vi "Teleop.vi"(10 "Match Info":T1={"Autonomous Elapsed Seconds"=0.0, "TeleOp Elapsed Seconds"=0.0, "Disabled Elapsed Seconds"=0.0, "Visited Autonomous"=FALSE, "Visited TeleOp"=FALSE, "Visited Disabled"=FALSE, "Autonomous Settings"={"Autonomous Style"=enum."Independent", "VI Refnum"=refnum}}, 11 "Call Context":T2) -> ()   [LabVIEW 2019]
doc: "This VI is called for each TeleOp packet received from the DS where the robot is not disabled. It is often used to read from the joysticks and update I/O or to update setpoints for timed control loops. It should complete and return within 20 milliseconds or it may miss DS packets."
uses:
  <vilib>/Rock Robotics/WPI/DriverStation/WPI_DriverStationDerivedRobotMode.ctl
  <vilib>/Rock Robotics/WPI/DriverStation/WPI_DriverStationMatch Info.ctl
  <vilib>/Rock Robotics/WPI/Utilities/WPI_GetSetVariantRefNum.vi
  Robot Global Data.vi
  <vilib>/Rock Robotics/Network Tables/NT Write Number.vi
  <vilib>/Rock Robotics/WPI/DriverStation/WPI_DriverStationRobotMode2.ctl
  <vilib>/Rock Robotics/Network Tables/NT Write Numeric Array.vi
  <vilib>/Rock Robotics/WPI/RobotDrive/WPI_RobotDriveArcadeDrive_Standard(NoSaturation).vi
  <vilib>/Rock Robotics/Network Tables/NT Write Boolean.vi
panel:
  in  "error in":errorcluster
  out "interpolation value":dbl format="%0.2f"
  # "Click here to set min"
  # "Click here to set max"
  # "Click here to set min"
  # "Click here to set max"
  # "Click here to set min"
  # "Click here to set max"
  # "Click here to set min"
  # "Click here to set max"
  # "Click here to set min"
  # "Click here to set max"
  # "Click here to set min"
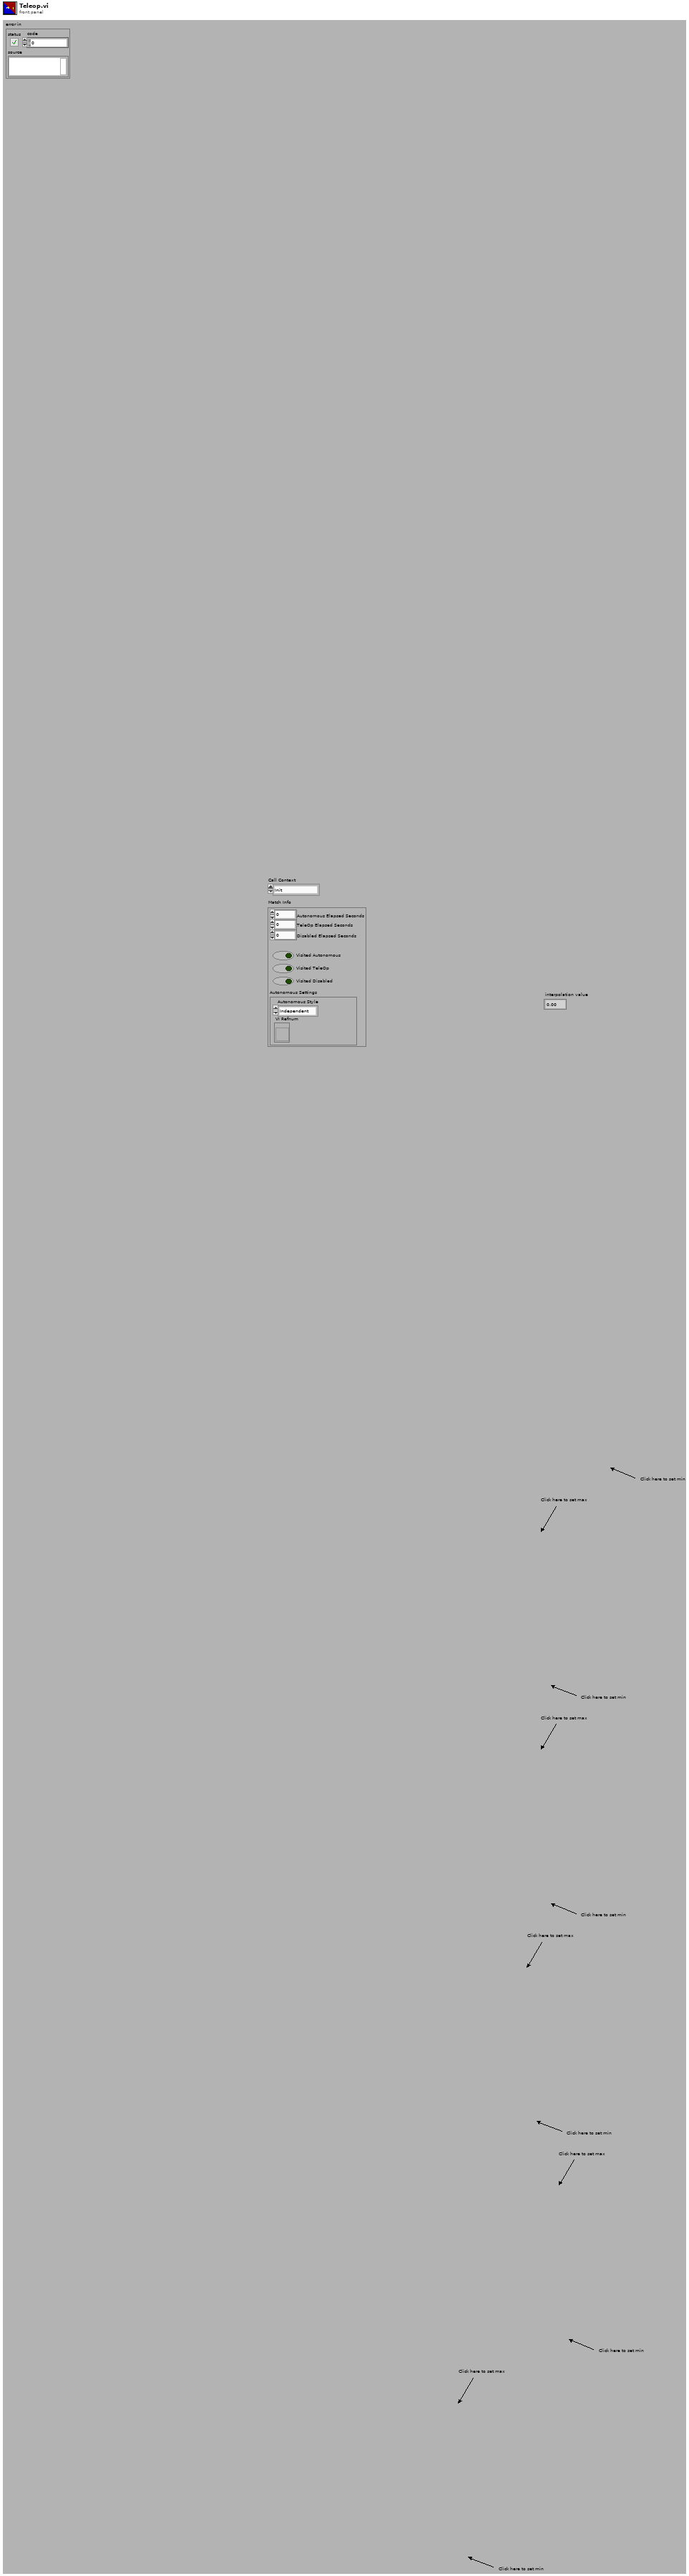
[diagram p1: front panel]
types:
  T1 = typedef "WPI_DriverStationMatch Info.ctl" = cluster{"Autonomous Elapsed Seconds":dbl, "TeleOp Elapsed Seconds":dbl, "Disabled Elapsed Seconds":dbl, "Visited Autonomous":bool, "Visited TeleOp":bool, "Visited Disabled":bool, "Autonomous Settings":cluster{"Autonomous Style":enum16{"Iterative", "Independent"}, "VI Refnum":refnum<vi>}}
  T2 = typedef "WPI_DriverStationDerivedRobotMode.ctl" = enum16{"Init", "Execute", "Stop"}
  T3 = typedef "WPI_JoystickDevRef.ctl" = cluster{"Device":T4}
  T4 = typedef "WPI_JoystickDeviceEnum.ctl" = enum16{"USB 0", "USB 1", "USB 2", "USB 3", "USB 4", "USB 5"}
  T5 = typedef "WPI_RobotDriveDevRef.ctl" = cluster{"DevStatus":errorcluster, "Motors[]":T6[], "Square Inputs":bool, "Max Output":dbl}
  T6 = typedef "WPI_MotorControlDeviceRef.ctl" = cluster{"DeviceStatus":errorcluster, "Type":T7, "PWM":cluster{"PWM Channel":T8, "DeadBand":T9}, "CAN":cluster{"Device Number":u8, "SetOutput VI Ref":variant, "GetOutput VI Ref":variant, "Enable VI Ref":variant, "Disable VI Ref":variant, "Data":variant}, "Invert":bool, "DIO PWM":cluster{"PWM \"Enable\" Channel":T8, "DIOChannel":T10, "PWM Rate":dbl}}
  T7 = typedef "WPI_MotorControlType.ctl" = enum16{"PWM", "CAN", "DIO PWM"}
  T8 = typedef "FPGA_DIOPWMChannel.ctl" = enum8{"PWM 0", "PWM 1", "PWM 2", "PWM 3", "PWM 4", "PWM 5", "PWM 6", "PWM 7", "PWM 8", "PWM 9", "PWM MXP 0", "PWM MXP 1", "PWM MXP 2", "PWM MXP 3", "PWM MXP 4", "PWM MXP 5", "PWM MXP 6", "PWM MXP 7", "PWM MXP 8", "PWM MXP 9", "Invalid"}
  T9 = typedef "WPI_PWMDeadband.ctl" = cluster{"Name":string, "maxPositivePwm":i32, "minPositivePwm":i32, "centerPwm":i32, "maxNegativePwm":i32, "minNegativePwm":i32, "angularRange":u16}
  T10 = typedef "FPGA_DIOChannel.ctl" = enum8{"DIO 0", "DIO 1", "DIO 2", "DIO 3", "DIO 4", "DIO 5", "DIO 6", "DIO 7", "DIO 8", "DIO 9", "DIO MXP 0", "DIO MXP 1", "DIO MXP 2", "DIO MXP 3", "DIO MXP 4", "DIO MXP 5", "DIO MXP 6", "DIO MXP 7", "DIO MXP 8", "DIO MXP 9", "DIO MXP 10", "DIO MXP 11", "DIO MXP 12", "DIO MXP 13", "DIO MXP 14", "DIO MXP 15", "SPI Port CS1", "SPI Port CS2", "SPI Port CS3", "SPI Port MISO", "SPI Port MOSI", "Invalid"}
  T11 = cluster{"JoystickDevRef":T3, "RobotDriveDevRef":T5}
  T12 = typedef "WPI_ServoDeviceRef.ctl" = cluster{"DeviceStatus":errorcluster, "PWM Channel":T8, "DeadBand":T9}
  T13 = typedef "WPI_DriverStationRobotMode2.ctl" = enum16{"Autonomous Disabled", "Autonomous Enabled", "Teleop Disabled", "Teleop Enabled", "Disconnected", "Finish", "Test Disabled", "Test Enabled", "Emergency Stopped"}
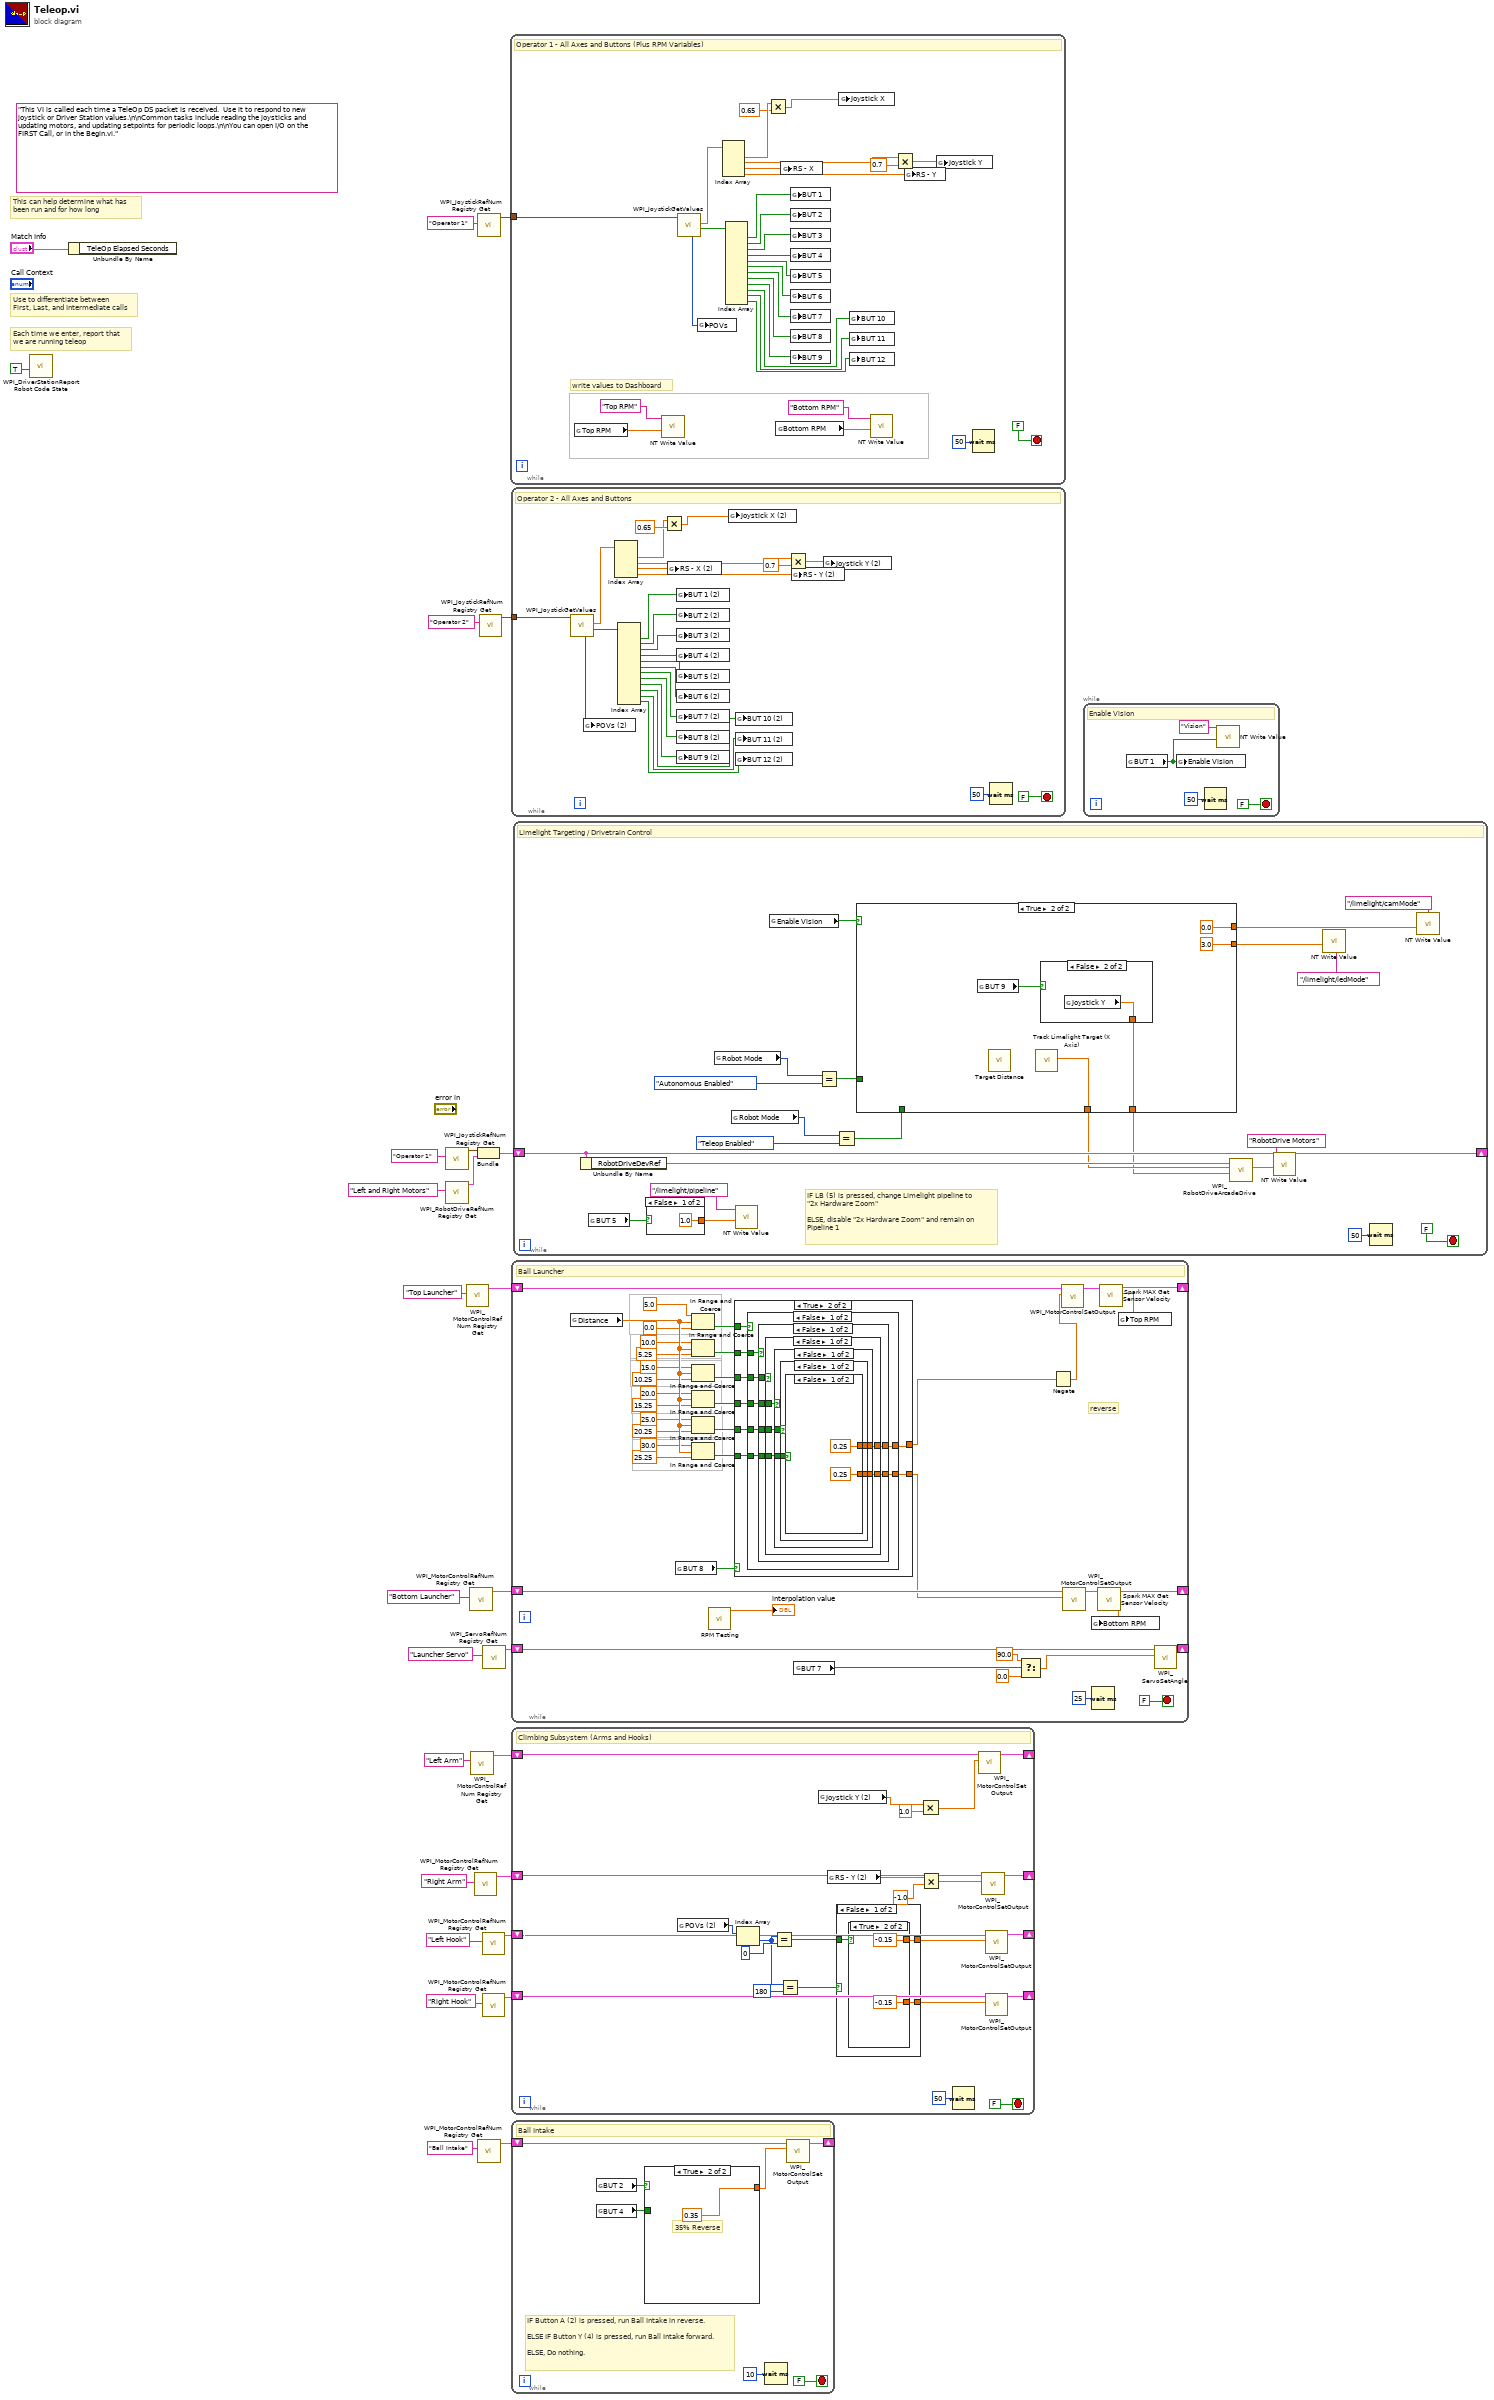
[diagram p0: block diagram]
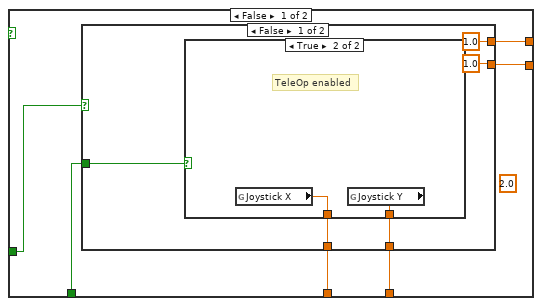
[diagram p2: hidden frame]
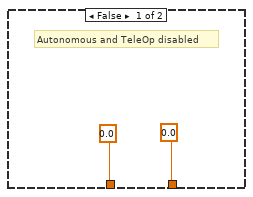
[diagram p3: hidden frame]
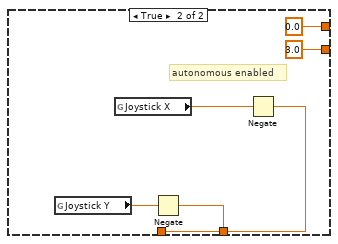
[diagram p4: hidden frame]
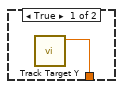
[diagram p5: hidden frame]
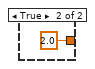
[diagram p6: hidden frame]
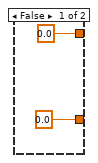
[diagram p7: hidden frame]
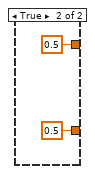
[diagram p8: hidden frame]
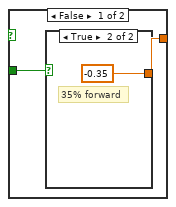
[diagram p9: hidden frame]
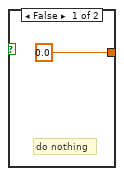
[diagram p10: hidden frame]
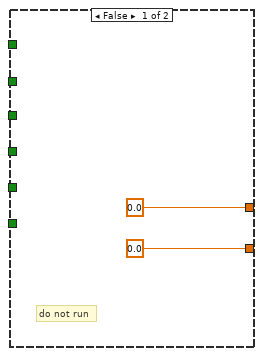
[diagram p11: hidden frame]
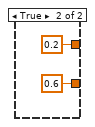
[diagram p12: hidden frame]
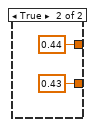
[diagram p13: hidden frame]
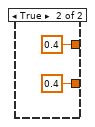
[diagram p14: hidden frame]
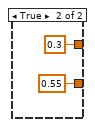
[diagram p15: hidden frame]
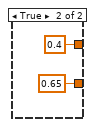
[diagram p16: hidden frame]
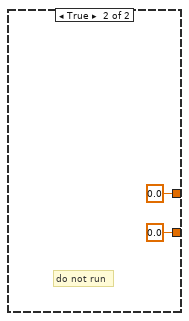
[diagram p17: hidden frame]
diagram:
  (unwired) "This VI is called each time a TeleOp DS packet is received.  Use it to respond to new joystick or Driver Station values.\n\nCommon tasks include reading the joysticks and updating motors, and updating setpoints for periodic loops.\n\nYou can open I/O on the FIRST Call, or in the Begin.vi."
  # "Each time we enter, report that\nwe are running teleop"
  # "Use to differentiate between\nFirst, Last, and Intermediate calls"
  # "This can help determine what has\nbeen run and for how long"
  n1 = call <vilib>:"WPI_DriverStationReport Robot Code State.vi"("TeleOp"=TRUE ("Autonomous")) -> ()  [unwired: 10 in, 1 out]
  n2 = Unbundle By Name("Match Info") -> ()  [unwired: 1 out]
  n3 = call <vilib>:"WPI_JoystickRefNum Registry Get.vi"("refnum name"="Operator 1") -> ("JoystickDevRef"=w3:T3)  [unwired: 1 in, 9 out]
  n4 = call <vilib>:"WPI_RobotDriveRefNum Registry Get.vi"("refnum name"="Left and Right Motors") -> ("RobotDriveDevRef"=w2:T5)  [unwired: 1 in, 9 out]
  n5 = call <vilib>:"WPI_MotorControlRefNum Registry Get.vi"("refnum name"="Top Launcher") -> ("MotorControlDevRef"=w21:T6)  [unwired: 9 in, 1 out]
  n6 = call <vilib>:"WPI_MotorControlRefNum Registry Get.vi"("refnum name"="Bottom Launcher") -> ("MotorControlDevRef"=w23:T6)  [unwired: 9 in, 1 out]
  n7 = call <vilib>:"WPI_MotorControlRefNum Registry Get.vi"("refnum name"="Left Arm") -> ("MotorControlDevRef"=w15:T6)  [unwired: 9 in, 1 out]
  n8 = call <vilib>:"WPI_MotorControlRefNum Registry Get.vi"("refnum name"="Right Arm") -> ("MotorControlDevRef"=w14:T6)  [unwired: 9 in, 1 out]
  n9 = Bundle("JoystickDevRef"=w3, "RobotDriveDevRef"=w2) -> (w1:T11)  [unwired: 1 out]
  n10 = call <vilib>:"WPI_JoystickRefNum Registry Get.vi"("refnum name"="Operator 1") -> ("JoystickDevRef"=w6:T3)  [unwired: 1 in, 9 out]
  n11 = call <vilib>:"WPI_MotorControlRefNum Registry Get.vi"("refnum name"="Ball Intake") -> ("MotorControlDevRef"=w17:T6)  [unwired: 9 in, 1 out]
  n12 = call <vilib>:"WPI_JoystickRefNum Registry Get.vi"("refnum name"="Operator 2") -> ("JoystickDevRef"=w7:T3)  [unwired: 1 in, 9 out]
  n13 = call <vilib>:"WPI_MotorControlRefNum Registry Get.vi"("refnum name"="Left Hook") -> ("MotorControlDevRef"=w12:T6)  [unwired: 9 in, 1 out]
  n14 = call <vilib>:"WPI_MotorControlRefNum Registry Get.vi"("refnum name"="Right Hook") -> ("MotorControlDevRef"=w11:T6)  [unwired: 9 in, 1 out]
  n15 = call <vilib>:"WPI_ServoRefNum Registry Get.vi"("refnum name"="Launcher Servo") -> ("ServoDeviceRef"=w19:T12)  [unwired: 9 in, 1 out]
  n16 = while {
    tunnel: w6 -> [w28]
    stop <- FALSE stop-if-true
    # "write values to Dashboard"
    # "Operator 1 - All Axes and Buttons (Plus RPM Variables)"
    n17 = global read "Robot Global Data.vi" "Top RPM"() -> (w39:dbl)
    n18 = call-poly <vilib>:"NT Write Value.vi"("Numeric"=w39, "Name"="Top RPM") -> ()  [unwired: 9 in, 1 out]
    n19 = call <vilib>:"WPI_JoystickGetValues.vi"("JoystickDevRef"=w28) -> ("Buttons"=w56:bool[], "Axes"=w43:dbl[], "POVs"=w35:i16[])  [unwired: 6 in, 2 out]
    n20 = global write "Robot Global Data.vi" "POVs"(w35) -> ()
    n21 = Index Array(array=w43) -> (element #1=w32:dbl, element #2=w34:dbl, element #3=w36:dbl, element #4=w42:dbl)  [unwired: 4 in]
    n22 = Index Array(array=w56) -> (element #1=w55:bool, element #2=w54:bool, element #3=w53:bool, element #4=w52:bool, element #5=w51:bool, element #6=w50:bool, element #7=w49:bool, element #8=w48:bool, element #9=w47:bool, element #10=w46:bool, element #11=w45:bool, element #12=w44:bool)  [unwired: 12 in]
    n23 = Multiply(x=w32, y=0.65) -> (x*y=w33:dbl)
    n24 = global read "Robot Global Data.vi" "Bottom RPM"() -> (w37:dbl)
    n25 = global write "Robot Global Data.vi" "RS - X"(w36) -> ()
    n26 = global write "Robot Global Data.vi" "BUT 1"(w55) -> ()
    n27 = global write "Robot Global Data.vi" "BUT 2"(w54) -> ()
    n28 = global write "Robot Global Data.vi" "BUT 3"(w53) -> ()
    n29 = global write "Robot Global Data.vi" "BUT 4"(w52) -> ()
    n30 = global write "Robot Global Data.vi" "BUT 5"(w51) -> ()
    n31 = global write "Robot Global Data.vi" "BUT 6"(w50) -> ()
    n32 = global write "Robot Global Data.vi" "BUT 7"(w49) -> ()
    n33 = global write "Robot Global Data.vi" "BUT 8"(w48) -> ()
    n34 = global write "Robot Global Data.vi" "BUT 9"(w47) -> ()
    n35 = global write "Robot Global Data.vi" "Joystick X"(w33) -> ()
    n36 = global write "Robot Global Data.vi" "BUT 10"(w46) -> ()
    n37 = global write "Robot Global Data.vi" "BUT 11"(w45) -> ()
    n38 = global write "Robot Global Data.vi" "BUT 12"(w44) -> ()
    n39 = call-poly <vilib>:"NT Write Value.vi"("Numeric"=w37, "Name"="Bottom RPM") -> ()  [unwired: 9 in, 1 out]
    n40 = Multiply(x=w34, y=0.7) -> (x*y=w30:dbl)
    n41 = global write "Robot Global Data.vi" "RS - Y"(w42) -> ()
    n42 = global write "Robot Global Data.vi" "Joystick Y"(w30) -> ()
    n43 = Wait (ms)(milliseconds to wait=u32 50) -> ()  [unwired: 1 out]
  }
  n44 = while {
    tunnel: w7 -> [w58]
    stop <- FALSE stop-if-true
    # "Operator 2 - All Axes and Buttons"
    n45 = call <vilib>:"WPI_JoystickGetValues.vi"("JoystickDevRef"=w58) -> ("Buttons"=w60:bool[], "Axes"=w73:dbl[], "POVs"=w59:i16[])  [unwired: 6 in, 2 out]
    n46 = global write "Robot Global Data.vi" "POVs (2)"(w59) -> ()
    n47 = Index Array(array=w73) -> (element #1=w78:dbl, element #2=w76:dbl, element #3=w75:dbl, element #4=w74:dbl)  [unwired: 4 in]
    n48 = Index Array(array=w60) -> (element #1=w61:bool, element #2=w62:bool, element #3=w63:bool, element #4=w64:bool, element #5=w65:bool, element #6=w66:bool, element #7=w67:bool, element #8=w68:bool, element #9=w69:bool, element #10=w70:bool, element #11=w71:bool, element #12=w72:bool)  [unwired: 12 in]
    n49 = Multiply(x=w78, y=0.65) -> (x*y=w77:dbl)
    n50 = global write "Robot Global Data.vi" "RS - X (2)"(w75) -> ()
    n51 = global write "Robot Global Data.vi" "BUT 1 (2)"(w61) -> ()
    n52 = global write "Robot Global Data.vi" "BUT 2 (2)"(w62) -> ()
    n53 = global write "Robot Global Data.vi" "BUT 3 (2)"(w63) -> ()
    n54 = global write "Robot Global Data.vi" "BUT 4 (2)"(w64) -> ()
    n55 = global write "Robot Global Data.vi" "BUT 5 (2)"(w65) -> ()
    n56 = global write "Robot Global Data.vi" "BUT 6 (2)"(w66) -> ()
    n57 = global write "Robot Global Data.vi" "BUT 7 (2)"(w67) -> ()
    n58 = global write "Robot Global Data.vi" "BUT 8 (2)"(w68) -> ()
    n59 = global write "Robot Global Data.vi" "BUT 9 (2)"(w69) -> ()
    n60 = global write "Robot Global Data.vi" "Joystick X (2)"(w77) -> ()
    n61 = global write "Robot Global Data.vi" "BUT 10 (2)"(w70) -> ()
    n62 = global write "Robot Global Data.vi" "BUT 11 (2)"(w71) -> ()
    n63 = global write "Robot Global Data.vi" "BUT 12 (2)"(w72) -> ()
    n64 = Multiply(x=w76, y=0.7) -> (x*y=w80:dbl)
    n65 = global write "Robot Global Data.vi" "RS - Y (2)"(w74) -> ()
    n66 = global write "Robot Global Data.vi" "Joystick Y (2)"(w80) -> ()
    n67 = Wait (ms)(milliseconds to wait=u32 50) -> ()  [unwired: 1 out]
  }
  n68 = while {
    shift-right: [w115] -> _
    shift-left: w23 -> [w116]
    shift-right: [w113] -> _
    shift-left: w21 -> [w114]
    shift-right: [w112] -> _
    shift-left: w19 -> [w107]
    stop <- FALSE stop-if-true
    # "reverse"
    # "Ball Launcher"
    n69 = global read "Robot Global Data.vi" "Distance"() -> (w105:dbl)
    n70 = global read "Robot Global Data.vi" "BUT 8"() -> (w86:bool)
    n71 = In Range and Coerce(upper limit=5.0, x=w105, lower limit=0.0) -> (In Range?=w104:bool)  [unwired: 1 out]
    n72 = In Range and Coerce(upper limit=10.0, x=w105, lower limit=5.25) -> (In Range?=w103:bool)  [unwired: 1 out]
    n73 = In Range and Coerce(upper limit=15.0, x=w105, lower limit=10.25) -> (In Range?=w87:bool)  [unwired: 1 out]
    n74 = In Range and Coerce(upper limit=20.0, x=w105, lower limit=15.25) -> (In Range?=w88:bool)  [unwired: 1 out]
    n75 = In Range and Coerce(upper limit=25.0, x=w105, lower limit=20.25) -> (In Range?=w89:bool)  [unwired: 1 out]
    n76 = In Range and Coerce(upper limit=30.0, x=w105, lower limit=25.25) -> (In Range?=w90:bool)  [unwired: 1 out]
    n77 = call "RPM Testing.vi"() -> ("interpolation value"=→"interpolation value":dbl)  [unwired: 11 in]
    n78 = case shown="True" w86 {
      tunnel: [0.0 ("Output") w127] -> w85
      tunnel: [0.0 ("Output") w126] -> w84
      tunnel: w104 -> [_ w133]
      tunnel: w87 -> [_ w131]
      tunnel: w88 -> [_ w130]
      tunnel: w89 -> [_ w129]
      tunnel: w90 -> [_ w128]
      tunnel: w103 -> [_ w132]
      frame False {
        # "do not run"
      }
      frame True {
        n79 = case shown="False" w133 {
          tunnel: w132 -> [w140 _]
          tunnel: w131 -> [w139 _]
          tunnel: w130 -> [w138 _]
          tunnel: w129 -> [w137 _]
          tunnel: w128 -> [w136 _]
          tunnel: [w135 0.0 ("Output")] -> w127
          tunnel: [w134 0.0 ("Output")] -> w126
          frame False {
            n80 = case shown="False" w140 {
              tunnel: w139 -> [w146 _]
              tunnel: w138 -> [w145 _]
              tunnel: w137 -> [w144 _]
              tunnel: w136 -> [w143 _]
              tunnel: [w142 0.4 ("Output")] -> w135
              tunnel: [w141 0.65 ("Output")] -> w134
              frame False {
                n81 = case shown="False" w146 {
                  tunnel: w145 -> [w151 _]
                  tunnel: w144 -> [w150 _]
                  tunnel: w143 -> [w149 _]
                  tunnel: [w148 0.3 ("Output")] -> w142
                  tunnel: [w147 0.55 ("Output")] -> w141
                  frame False {
                    n82 = case shown="False" w151 {
                      tunnel: w150 -> [w155 _]
                      tunnel: w149 -> [w154 _]
                      tunnel: [w153 0.4 ("Output")] -> w148
                      tunnel: [w152 0.4 ("Output")] -> w147
                      frame False {
                        n83 = case shown="False" w155 {
                          tunnel: w154 -> [w158 _]
                          tunnel: [w157 0.44 ("Output")] -> w153
                          tunnel: [w156 0.43 ("Output")] -> w152
                          frame False {
                            n84 = case shown="False" w158 {
                              tunnel: [0.25 ("Output") 0.2 ("Output")] -> w157
                              tunnel: [0.25 ("Output") 0.6 ("Output")] -> w156
                              frame False {
                              }
                              frame True {
                              }
                            }
                          }
                          frame True {
                          }
                        }
                      }
                      frame True {
                      }
                    }
                  }
                  frame True {
                  }
                }
              }
              frame True {
              }
            }
          }
          frame True {
            # "do not run"
          }
        }
      }
    }
    n85 = global read "Robot Global Data.vi" "BUT 7"() -> (w111:bool)
    n86 = Select(t=90.0, s=w111, f=0.0) -> (s? t:f=w108:dbl)
    n87 = Negate(x=w85) -> (-x=w123:dbl)
    n88 = call <vilib>:"WPI_MotorControlSetOutput.vi"("Output"=w123, "MotorControlDevRef"=w114) -> ("MotorControlDevRef"=w121:T6)  [unwired: 7 in, 2 out]
    n89 = call <vilib>:"WPI_MotorControlSetOutput.vi"("Output"=w84, "MotorControlDevRef"=w116) -> ("MotorControlDevRef"=w122:T6)  [unwired: 7 in, 2 out]
    n90 = Wait (ms)(milliseconds to wait=u32 25) -> ()  [unwired: 1 out]
    n91 = call <vilib>:"Spark MAX Get Sensor Velocity.vi"("MotorControlDevRef in"=w122) -> ("Sensor Velocity"=w120:dbl, "MotorControlDevRef out"=w115:T6)  [unwired: 7 in, 2 out]
    n92 = global write "Robot Global Data.vi" "Bottom RPM"(w120) -> ()
    n93 = call <vilib>:"Spark MAX Get Sensor Velocity.vi"("MotorControlDevRef in"=w121) -> ("Sensor Velocity"=w119:dbl, "MotorControlDevRef out"=w113:T6)  [unwired: 7 in, 2 out]
    n94 = global write "Robot Global Data.vi" "Top RPM"(w119) -> ()
    n95 = call <vilib>:"WPI_ServoSetAngle.vi"("Angle"=w108, "ServoDeviceRef"=w107) -> ("ServoDeviceRef"=w112:T12)  [unwired: 8 in, 1 out]
  }
  n96 = while {
    shift-right: [w195] -> _
    shift-left: w15 -> [w194]
    shift-right: [w192] -> _
    shift-left: w14 -> [w193]
    shift-right: [w185] -> _
    shift-left: w11 -> [w184]
    shift-right: [w186] -> _
    shift-left: w12 -> [w183]
    stop <- FALSE stop-if-true
    # "Climbing Subsystem (Arms and Hooks)"
    n97 = global read "Robot Global Data.vi" "POVs (2)"() -> (w191:i16[])
    n98 = Index Array(array=w191) -> (element=w189:i16)  [unwired: 1 in]
    n99 = Equal?(x=w189, y=i16 0) -> (x = y?=w173:bool)
    n100 = Equal?(x=w189, y=i16 180) -> (x = y?=w174:bool)
    n101 = global read "Robot Global Data.vi" "Joystick Y (2)"() -> (w180:dbl)
    n102 = global read "Robot Global Data.vi" "RS - Y (2)"() -> (w177:dbl)
    n103 = case shown="False" w174 {
      tunnel: [w199 0.5 ("Output")] -> w176
      tunnel: [w198 0.5 ("Output")] -> w175
      tunnel: w173 -> [w197 _]
      frame False {
        n104 = case shown="True" w197 {
          tunnel: [0.0 ("Output") -0.15 ("Output")] -> w199
          tunnel: [0.0 ("Output") -0.15 ("Output")] -> w198
          frame False {
          }
          frame True {
          }
        }
      }
      frame True {
      }
    }
    n105 = Multiply(x=w180, y=1.0) -> (x*y=w182:dbl)
    n106 = Multiply(x=w177, y=-1.0) -> (x*y=w181:dbl)
    n107 = Wait (ms)(milliseconds to wait=u32 50) -> ()  [unwired: 1 out]
    n108 = call <vilib>:"WPI_MotorControlSetOutput.vi"("Output"=w182, "MotorControlDevRef"=w194) -> ("MotorControlDevRef"=w195:T6)  [unwired: 7 in, 2 out]
    n109 = call <vilib>:"WPI_MotorControlSetOutput.vi"("Output"=w181, "MotorControlDevRef"=w193) -> ("MotorControlDevRef"=w192:T6)  [unwired: 7 in, 2 out]
    n110 = call <vilib>:"WPI_MotorControlSetOutput.vi"("Output"=w175, "MotorControlDevRef"=w183) -> ("MotorControlDevRef"=w186:T6)  [unwired: 7 in, 2 out]
    n111 = call <vilib>:"WPI_MotorControlSetOutput.vi"("Output"=w176, "MotorControlDevRef"=w184) -> ("MotorControlDevRef"=w185:T6)  [unwired: 7 in, 2 out]
  }
  n112 = while {
    shift-right: [w209] -> _
    shift-left: w17 -> [w210]
    stop <- FALSE stop-if-true
    # "IF Button A (2) is pressed, run Ball Intake in reverse. \n\nELSE IF Button Y (4) is pressed, run Ball Intake forward.\n\nELSE, Do nothing."
    # "Ball Intake"
    n113 = global read "Robot Global Data.vi" "BUT 2"() -> (w207:bool)
    n114 = global read "Robot Global Data.vi" "BUT 4"() -> (w208:bool)
    n115 = case shown="True" w207 {
      tunnel: [w214 0.35 ("Output")] -> w206
      tunnel: w208 -> [w213 _]
      frame False {
        n116 = case shown="True" w213 {
          tunnel: [0.0 ("Output") -0.35 ("Output")] -> w214
          frame False {
            # "do nothing"
          }
          frame True {
            # "35% forward"
          }
        }
      }
      frame True {
        # "35% Reverse"
      }
    }
    n117 = Wait (ms)(milliseconds to wait=u32 10) -> ()  [unwired: 1 out]
    n118 = call <vilib>:"WPI_MotorControlSetOutput.vi"("Output"=w206, "MotorControlDevRef"=w210) -> ("MotorControlDevRef"=w209:T6)  [unwired: 7 in, 2 out]
  }
  n119 = while {
    shift-right: [w238] -> _
    shift-left: w1 -> [w238]
    stop <- FALSE stop-if-true
    # "IF LB (5) is pressed, change Limelight pipeline to \n\"2x Hardware Zoom\"\n\nELSE, disable \"2x Hardware Zoom\" and remain on\nPipeline 1"
    # "Limelight Targeting / Drivetrain Control"
    n120 = Unbundle By Name(w238) -> ("RobotDriveDevRef"=w235:T5)
    n121 = global read "Robot Global Data.vi" "BUT 5"() -> (w220:bool)
    n122 = case shown="False" w220 {
      tunnel: [1.0 ("Numeric") 2.0 ("Numeric")] -> w234
      frame False {
      }
      frame True {
      }
    }
    n123 = global read "Robot Global Data.vi" "Robot Mode"() -> (w229:T13)
    n124 = global read "Robot Global Data.vi" "Robot Mode"() -> (w225:T13)
    n125 = call-poly <vilib>:"NT Write Value.vi"("Numeric"=w234, "Name"="/limelight/pipeline") -> ()  [unwired: 9 in, 1 out]
    n126 = global read "Robot Global Data.vi" "Enable Vision"() -> (w221:bool)
    n127 = Equal?(x=w229, y=WPI_DriverStationRobotMode2."Autonomous Enabled") -> (x = y?=w227:bool)
    n128 = Equal?(x=w225, y=WPI_DriverStationRobotMode2."Teleop Enabled") -> (x = y?=w224:bool)
    n129 = case shown="True" w221 {
      tunnel: [w242 0.0 ("Numeric")] -> w231
      tunnel: [w241 3.0 ("Numeric")] -> w230
      tunnel: [w245 w263] -> w222
      tunnel: w227 -> [w243 _]
      tunnel: w224 -> [w244 _]
      tunnel: [w240 w262] -> w223
      frame False {
        (unwired) 2.0 ("Numeric")
        n130 = case shown="False" w243 {
          tunnel: [w249 w259] -> w245
          tunnel: [w250 w258] -> w240
          tunnel: w244 -> [w248 _]
          tunnel: [1.0 ("Numeric") 0.0 ("Numeric")] -> w242
          tunnel: [1.0 ("Numeric") 3.0 ("Numeric")] -> w241
          frame False {
            n131 = case shown="True" w248 {
              tunnel: [0.0 ("Joystick X") w254] -> w250
              tunnel: [0.0 ("Joystick Y") w253] -> w249
              frame False {
                # "Autonomous and TeleOp disabled"
              }
              frame True {
                # "TeleOp enabled"
                n132 = global read "Robot Global Data.vi" "Joystick X"() -> (w254:dbl)
                n133 = global read "Robot Global Data.vi" "Joystick Y"() -> (w253:dbl)
              }
            }
          }
          frame True {
            # "autonomous enabled"
            n134 = global read "Robot Global Data.vi" "Joystick Y"() -> (w260:dbl)
            n135 = global read "Robot Global Data.vi" "Joystick X"() -> (w257:dbl)
            n136 = Negate(x=w260) -> (-x=w259:dbl)
            n137 = Negate(x=w257) -> (-x=w258:dbl)
          }
        }
      }
      frame True {
        n138 = global read "Robot Global Data.vi" "BUT 9"() -> (w261:bool)
        n139 = call "Target Distance.vi"() -> ()  [unwired: 12 in]
        n140 = call "Track Limelight Target (X Axis).vi"() -> ("Joystick X"=w262:dbl)  [unwired: 11 in]
        n141 = case shown="False" w261 {
          tunnel: [w266 w267] -> w263
          frame True {
            n142 = call "Track Target Y.vi"() -> ("Joystick Y"=w266:dbl)  [unwired: 11 in]
          }
          frame False {
            n143 = global read "Robot Global Data.vi" "Joystick Y"() -> (w267:dbl)
          }
        }
      }
    }
    n144 = call-poly <vilib>:"WPI_RobotDriveArcadeDrive.vi"("Y axis value"=w222, "X axis value"=w223, "RobotDriveDevRef"=w235) -> ("Motor Values"=w218:dbl[])  [unwired: 6 in, 2 out]
    n145 = call-poly <vilib>:"NT Write Value.vi"("Numeric Array"=w218, "Name"="RobotDrive Motors") -> ()  [unwired: 9 in, 1 out]
    n146 = call-poly <vilib>:"NT Write Value.vi"("Numeric"=w230, "Name"="/limelight/ledMode" ("LED Mode")) -> ()  [unwired: 9 in, 1 out]
    n147 = Wait (ms)(milliseconds to wait=u32 50) -> ()  [unwired: 1 out]
    n148 = call-poly <vilib>:"NT Write Value.vi"("Numeric"=w231, "Name"="/limelight/camMode" ("Camera Mode")) -> ()  [unwired: 9 in, 1 out]
  }
  n149 = while {
    stop <- FALSE stop-if-true
    # "Enable Vision"
    n150 = global read "Robot Global Data.vi" "BUT 1"() -> (w270:bool)
    n151 = global write "Robot Global Data.vi" "Enable Vision"(w270) -> ()
    n152 = Wait (ms)(milliseconds to wait=u32 50) -> ()  [unwired: 1 out]
    n153 = call-poly <vilib>:"NT Write Value.vi"("Boolean"=w270, "Name"="Vision") -> ()  [unwired: 9 in, 1 out]
  }
